vi "数据查询.vi"() -> ()   [LabVIEW 2016, in "数据查询.lvlib"]
uses:
  <vilib>/Utility/sysdir.llb/System Directory Type.ctl
  <vilib>/Utility/miscctls.llb/LVPointTypeDef.ctl
  var/holding var.vi
  <vilib>/ptbypt/NI_PtbyPt.lvlib
panel:
  out "布尔":bool
  in  "设置按钮":bool
  in  "标识说明":bool
  in  "数据查询菜单":enum32{"数据查询", "仪器数据", "仪器日志", "报警信息", "校准日志"}(xcontrol)
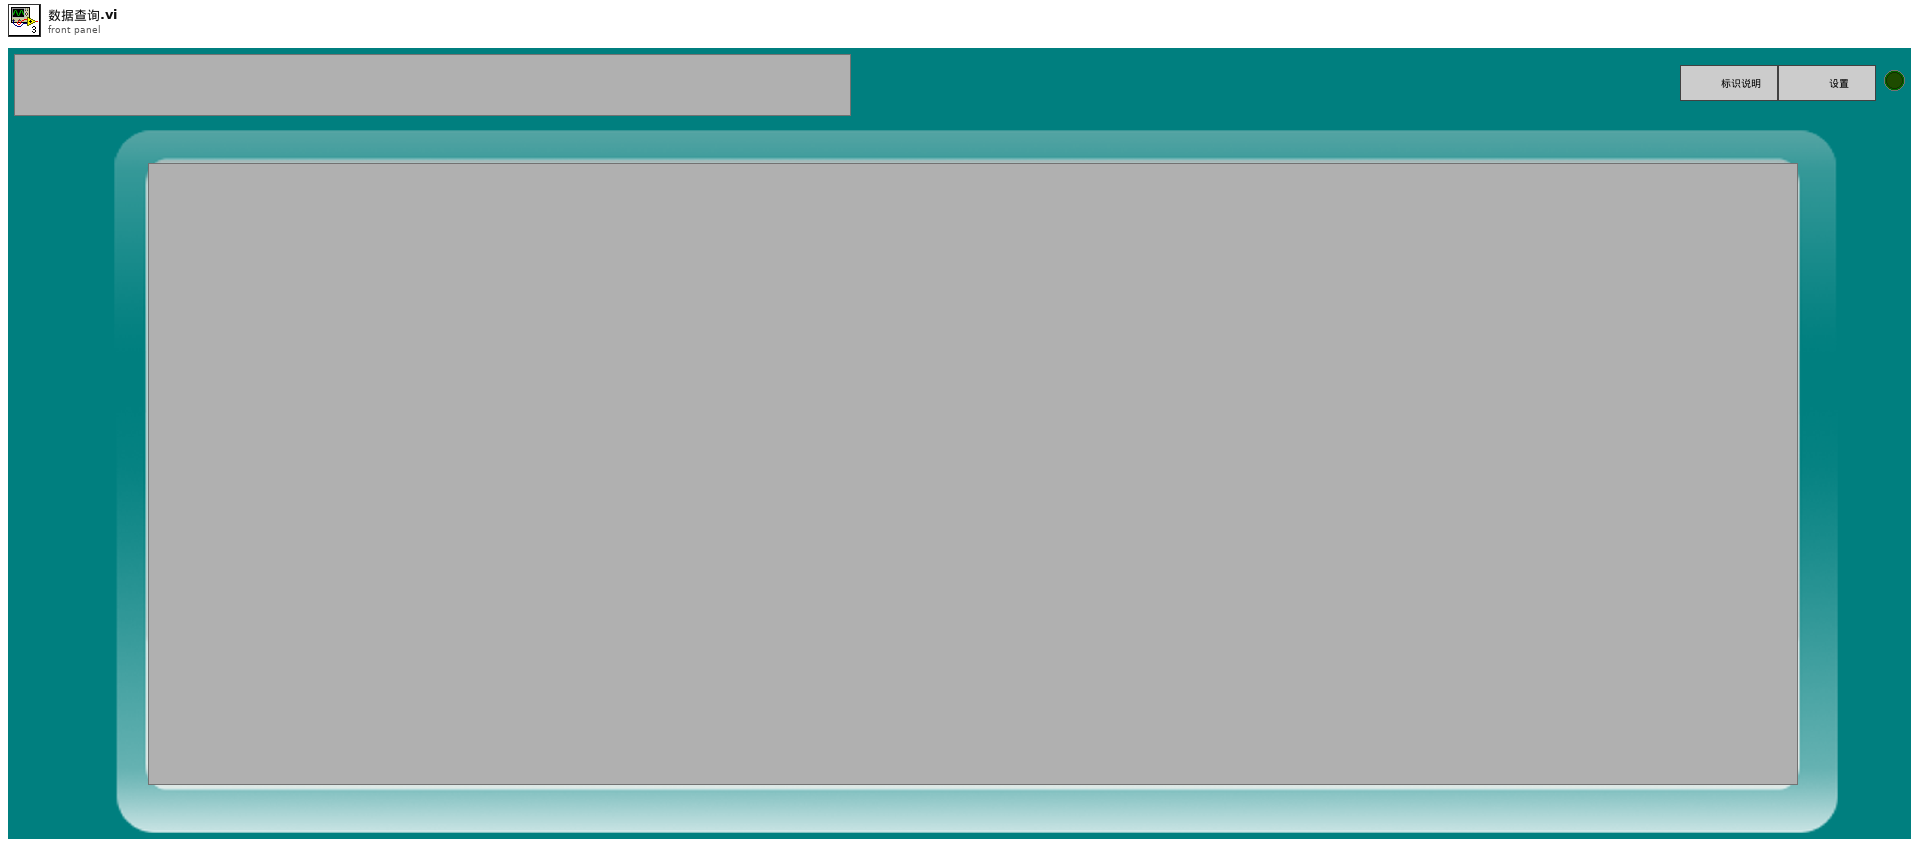
[diagram p1: front panel]
types:
  T1 = typedef "LVPointTypeDef.ctl" = cluster{"Horizontal":i16, "Vertical":i16}
  T2 = typedef "LVDateTimeRec.ctl" = cluster{"秒数的小数部分":dbl, "秒":i32, "分":i32, "时":i32, "日":i32, "月":i32, "年":i32, "天数（周）":i32, "天数（年）":i32, "DST":i32}
  T3 = typedef "System Directory Type.ctl" = i32
  T4 = enum32{"Bad", "Idle", "Run top level", "Running"}
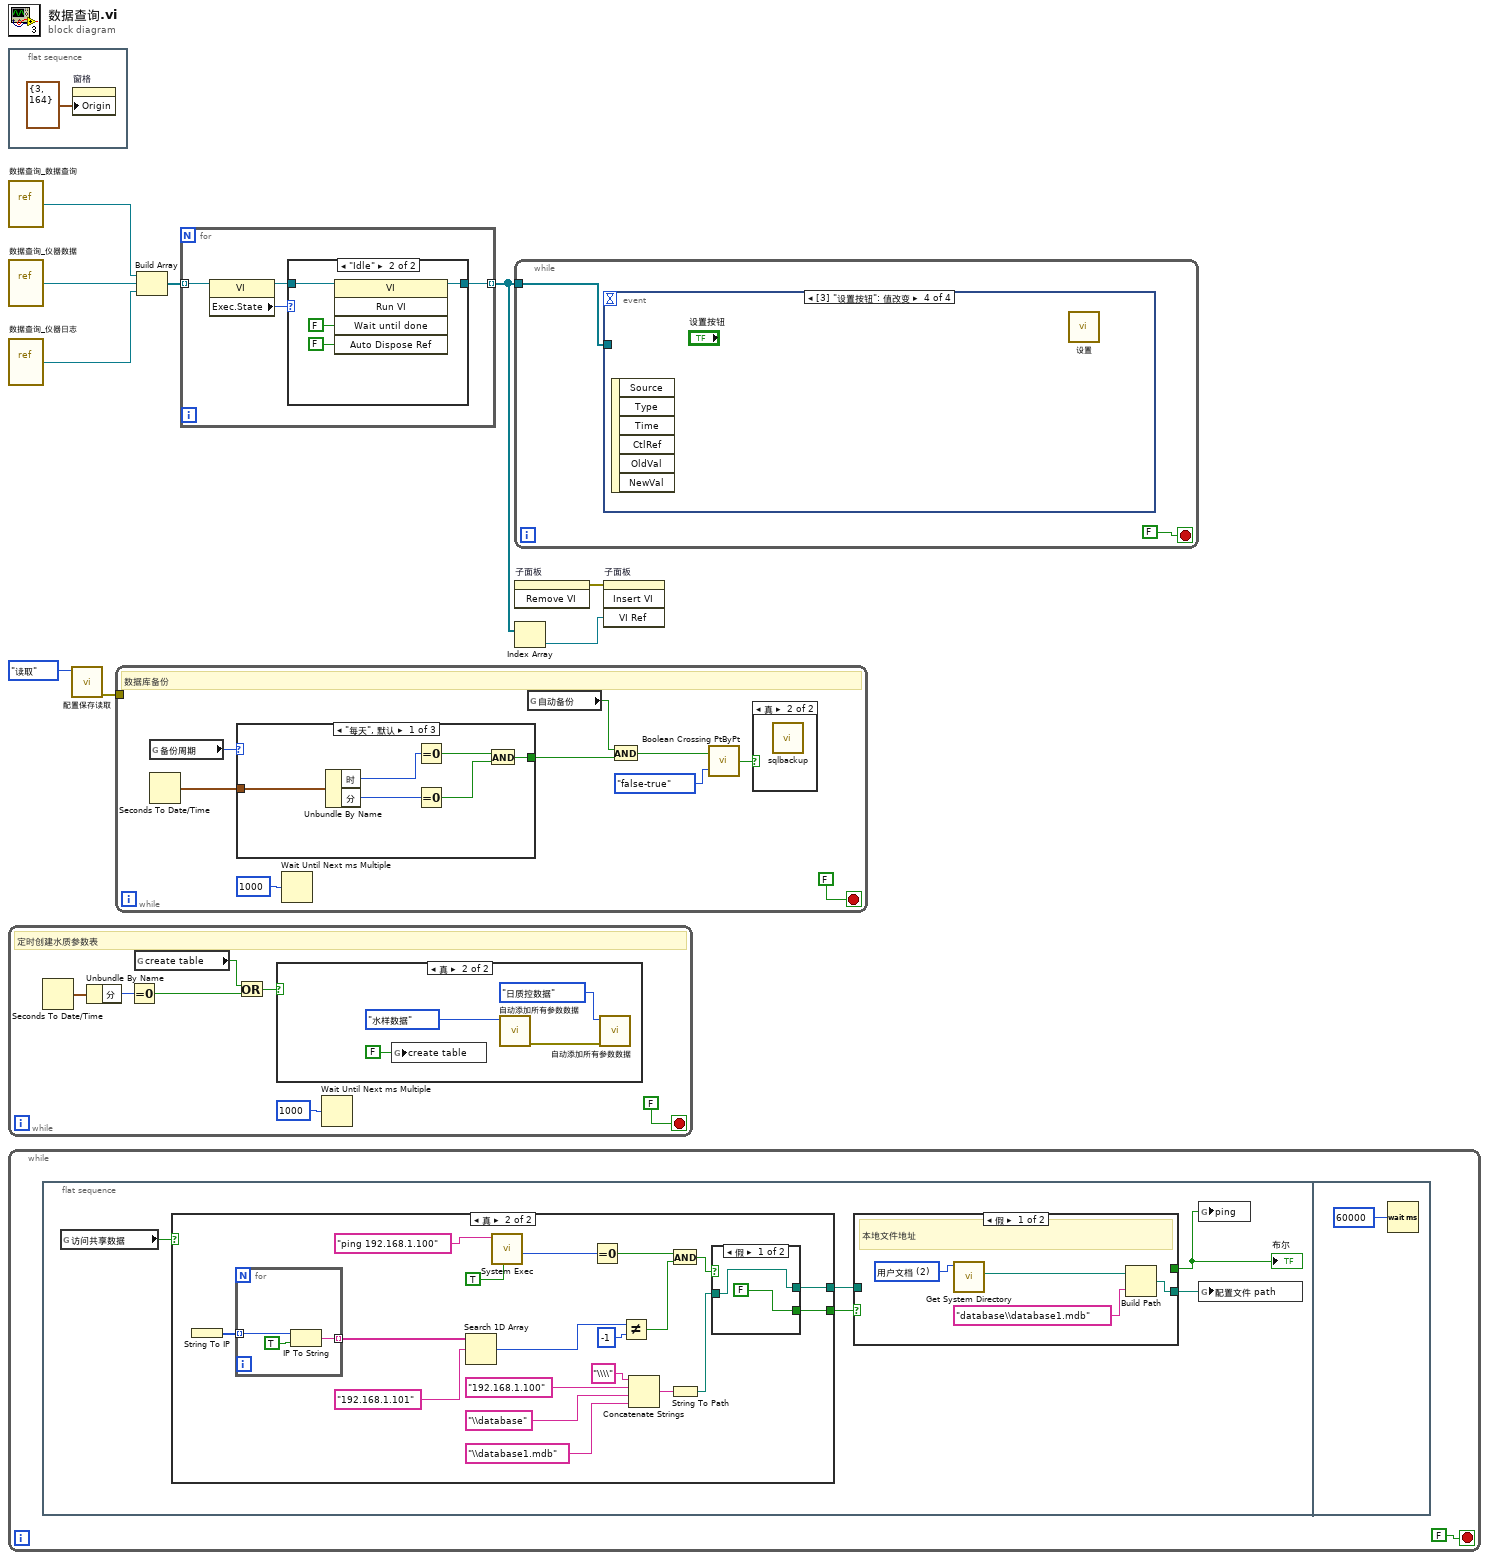
[diagram p0: block diagram]
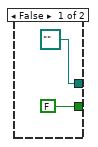
[diagram p2: hidden frame]
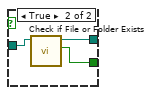
[diagram p3: hidden frame]
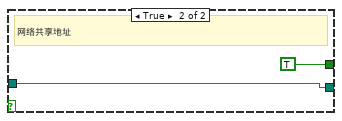
[diagram p4: hidden frame]
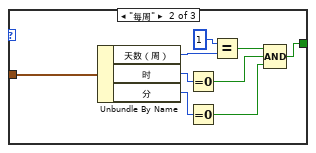
[diagram p6: hidden frame]
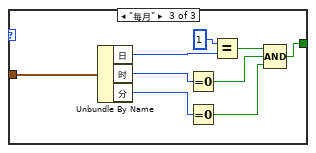
[diagram p7: hidden frame]
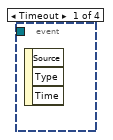
[diagram p10: hidden frame]
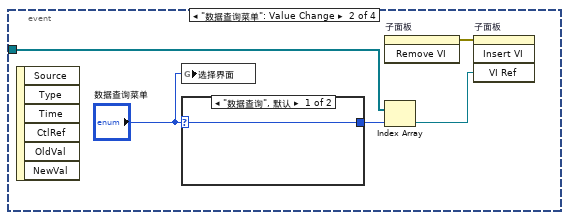
[diagram p11: hidden frame]
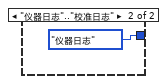
[diagram p12: hidden frame]
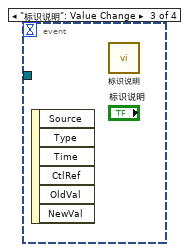
[diagram p13: hidden frame]
diagram:
  n1 = flat-sequence {
    frame #0 {
      n2 = property on="窗格" class="Pane"("Origin"=T1 {"Horizontal"=3, "Vertical"=164} ("原点")) -> ()  [unwired: 2 in, 2 out]
    }
  }
  n3 = vi-ref "数据查询_数据查询.vi"() -> (w6:refnum<vi>)
  n4 = vi-ref "数据查询_仪器数据.vi"() -> (w4:refnum<vi>)
  n5 = vi-ref "数据查询_仪器日志.vi"() -> (w3:refnum<vi>)
  n6 = while {
    stop <- FALSE stop-if-true
    # "定时创建水质参数表"
    n7 = Seconds To Date/Time() -> (date time rec=w17:T2)  [unwired: 2 in]
    n8 = Unbundle By Name(w17) -> ("分"=w16:i32)
    n9 = Equal To 0?(x=w16) -> (x = 0?=w13:bool)
    n10 = global read "全局变量.vi" "create table"() -> (w12:bool)
    n11 = Or(x=w12, y=w13) -> (x .or. y?=w14:bool)
    n12 = case shown="真" w14 {
      frame False {
      }
      frame True {
        n13 = global write "全局变量.vi" "create table"(FALSE ("create table")) -> ()
        n14 = call "自动添加所有参数数据.vi"("数据类别"=enum16{"水样数据", "日质控数据"}."水样数据") -> ("错误输出"=w21:errorcluster)  [unwired: 10 in]
        n15 = call "自动添加所有参数数据.vi"("error in (no error)"=w21, "数据类别"=enum16{"水样数据", "日质控数据"}."日质控数据") -> ()  [unwired: 9 in, 1 out]
      }
    }
    n16 = Wait Until Next ms Multiple(millisecond multiple=u32 1000 ("毫秒倍数")) -> ()  [unwired: 1 out]
  }
  n17 = while {
    stop <- FALSE stop-if-true
    n18 = flat-sequence {
      frame #0 {
        n19 = global read "全局变量.vi" "访问共享数据"() -> (w24:bool)
        n20 = case shown="真" w24 {
          tunnel: [path "" ("dup path") w42] -> w27
          tunnel: [FALSE ("file or folder exists?") w41] -> w26
          frame False {
          }
          frame True {
            n21 = String To IP() -> (0:w35:u32[])  [unwired: 1 in]
            n22 = for {
              tunnel: w35 -> [w51] mode=indexing
              tunnel: [w50] -> w34 mode=indexing
              n23 = IP To String(1:TRUE ("句点符号？(F)"), 2:w51) -> (0:w50:string)
            }
            n24 = Search 1D Array(1D array=w34, element="192.168.1.101" ("command line")) -> (index of element=w32:i32)  [unwired: 1 in]
            n25 = call <vilib>:"System Exec.vi"("run minimized? (F)"=TRUE, "command line"="ping 192.168.1.100") -> ("return code"=w38:i32)  [unwired: 6 in, 3 out]
            n26 = Equal To 0?(x=w38) -> (x = 0?=w37:bool)
            n27 = Not Equal?(x=w32, y=-1) -> (x != y?=w30:bool)
            n28 = Concatenate Strings("\\\\" ("字符串"), "192.168.1.100" ("名称"), "\\database" ("字符串"), "\\database1.mdb" ("名称或相对路径")) -> (w47:string)
            n29 = And(x=w37, y=w30) -> (x .and. y?=w36:bool)
            n30 = String To Path(string=w47) -> (path=w44:path)
            n31 = case shown="假" w36 {
              tunnel: w44 -> [w52 w56]
              tunnel: [w52 w55] -> w42
              tunnel: [FALSE w54] -> w41
              frame False {
              }
              frame True {
                n32 = call <vilib>:"Check if File or Folder Exists.vi"("path"=w56) -> ("file or folder exists?"=w54:bool, "dup path"=w55:path)  [unwired: 8 in, 1 out]
              }
            }
          }
        }
        n33 = case shown="假" w26 {
          tunnel: w27 -> [_ w62]
          tunnel: [w59 w62] -> w25
          tunnel: [_ TRUE] -> w23
          frame False {
            w57 = T3 2 items=["用户目录"=0, "用户桌面"=1, "用户文档"=2, "用户应用程序数据"=3, "用户设置"=4, "用户临时目录"=5, "公共文档"=6, "公共应用程序数据"=7, "公共设置"=8, "公共缓存"=13, "系统核心库"=9, "系统安装库"=10, "应用程序文件"=11, "启动盘根目录"=12] ("system directory type")
            # "本地文件地址"
            n34 = call <vilib>:"Get System Directory.vi"("system directory type"=w57) -> ("system directory"=w58:path)  [unwired: 10 in]
            n35 = Build Path(base path=w58, name or relative path="database\\database1.mdb" ("名称或相对路径")) -> (appended path=w59:path)
          }
          frame True {
            # "网络共享地址"
          }
        }
        "布尔" <- w23
        n36 = global write "全局变量.vi" "ping"(w23) -> ()
        n37 = global write "全局变量.vi" "配置文件 path"(w25) -> ()
      }
      frame #1 {
        n38 = Wait (ms)(milliseconds to wait=u32 60000 ("等待时间（毫秒）")) -> ()  [unwired: 1 out]
      }
    }
  }
  n39 = call "配置保存读取.vi"("配置"=enum16{"读取", "写入"}."读取") -> ("error out"=w1:errorcluster)  [unwired: 10 in]
  n40 = while {
    tunnel: w1 -> [_]
    stop <- FALSE stop-if-true
    # "数据库备份"
    n41 = global read "holding var.vi" "备份周期"() -> (w71:enum16{"每天", "每周", "每月"})
    n42 = Seconds To Date/Time() -> (date time rec=w66:T2)  [unwired: 2 in]
    n43 = case shown="\"每天\", 默认" w71 {
      tunnel: w66 -> [w78 w87 w96]
      tunnel: [w73 w79 w88] -> w65
      frame "每天", Default {
        n44 = Unbundle By Name(w78) -> ("时"=w76:i32, "分"=w77:i32)
        n45 = Equal To 0?(x=w76) -> (x = 0?=w74:bool)
        n46 = Equal To 0?(x=w77) -> (x = 0?=w75:bool)
        n47 = And(x=w74, y=w75) -> (x .and. y?=w73:bool)
      }
      frame "每周" {
        n48 = Unbundle By Name(w87) -> ("天数（周）"=w86:i32, "时"=w84:i32, "分"=w83:i32)
        n49 = Equal To 0?(x=w84) -> (x = 0?=w81:bool)
        n50 = Equal To 0?(x=w83) -> (x = 0?=w80:bool)
        n51 = Equal?(x=1, y=w86) -> (x = y?=w82:bool)
        n52 = Compound Arithmetic op=AND ("复合运算")(w82, w81, w80) -> (w79:bool)
      }
      frame "每月" {
        n53 = Unbundle By Name(w96) -> ("日"=w95:i32, "时"=w93:i32, "分"=w92:i32)
        n54 = Equal To 0?(x=w93) -> (x = 0?=w90:bool)
        n55 = Equal To 0?(x=w92) -> (x = 0?=w89:bool)
        n56 = Equal?(x=1, y=w95) -> (x = y?=w91:bool)
        n57 = Compound Arithmetic op=AND ("复合运算")(w91, w90, w89) -> (w88:bool)
      }
    }
    n58 = Wait Until Next ms Multiple(millisecond multiple=u32 1000 ("毫秒倍数")) -> ()  [unwired: 1 out]
    n59 = global read "holding var.vi" "自动备份"() -> (w70:bool)
    n60 = And(x=w70, y=w65) -> (x .and. y?=w69:bool)
    n61 = call <vilib>:"Boolean Crossing PtByPt.vi"("direction"=enum16{"either", "false-true", "true-false"}."false-true", "input"=w69) -> ("crossing"=w67:bool)  [unwired: 1 in]
    n62 = case shown="真" w67 {
      frame False {
      }
      frame True {
        n63 = call "sqlbackup.vi"() -> ()  [unwired: 11 in, 1 out]
      }
    }
  }
  n64 = Build Array(w6, w4, w3) -> (w5:refnum<vi>[])
  n65 = for {
    tunnel: w5 -> [w100] mode=indexing
    tunnel: [w97] -> w8 mode=indexing
    n66 = property class="VI"(reference=w100) -> (reference out=w98:refnum<vi>, "Exec.State"=w99:T4)  [unwired: 1 in, 1 out]
    n67 = case shown="\"Idle\"" w99 {
      tunnel: w98 -> [w101 w103]
      tunnel: [w101 w102] -> w97
      frame "Bad", Default {
      }
      frame "Idle" {
        n68 = invoke class="VI" method="Run VI"(reference=w103, "Wait until done"=FALSE ("结束前等待"), "Auto Dispose Ref"=FALSE ("自动销毁引用")) -> (reference out=w102:refnum<vi>)  [unwired: 2 in, 4 out]
      }
    }
  }
  n69 = while {
    tunnel: w8 -> [w106]
    stop <- FALSE stop-if-true
    n70 = event shown="[3] \"设置按钮\": 值改变" {
      selector: _ -> [_ _ _ _]
      dyn-events: _ -> [_ _ _ _]
      timeout: _ -> [_ _ _ _]
      tunnel: w106 -> [_ w112 _ _]
      event Timeout {
        n71 = event-data() -> ()  [unwired: 1 in, 3 out]
      }
      event "数据查询菜单": Value Change {
        n72 = event-data() -> ()  [unwired: 1 in, 6 out]
        n73 = global write "全局变量.vi" "选择界面"("数据查询菜单") -> ()
        n74 = case shown="\"数据查询\", 默认" "数据查询菜单" {
          selector: "数据查询菜单" -> [w113 _]
          tunnel: [w113 enum32{"数据查询", "仪器数据", "仪器日志", "报警信息", "校准日志"}."仪器日志" ("数据查询菜单")] -> w109
          frame "数据查询", Default {
          }
          frame "仪器日志".."校准日志" {
          }
        }
        n75 = invoke on="子面板" class="SubPnl" method="Remove VI"() -> (error out=w110:errorcluster)  [unwired: 3 in, 2 out]
        n76 = Index Array(array=w112, index=w109) -> (element=w111:refnum<vi>)
        n77 = invoke on="子面板" class="SubPnl" method="Insert VI"(error in=w110, "VI Ref"=w111) -> ()  [unwired: 2 in, 4 out]
      }
      event "标识说明": Value Change {
        n78 = event-data() -> ()  [unwired: 1 in, 6 out]
        n79 = call "标识说明.vi"() -> ()  [unwired: 12 in]
      }
      event "设置按钮": Value Change {
        n80 = event-data() -> ()  [unwired: 1 in, 6 out]
        n81 = call "设置.vi"() -> ()  [unwired: 12 in]
      }
    }
  }
  n82 = invoke on="子面板" class="SubPnl" method="Remove VI"() -> (error out=w9:errorcluster)  [unwired: 3 in, 2 out]
  n83 = Index Array(array=w8) -> (element=w7:refnum<vi>)  [unwired: 1 in]
  n84 = invoke on="子面板" class="SubPnl" method="Insert VI"(error in=w9, "VI Ref"=w7) -> ()  [unwired: 2 in, 4 out]
